vi "CNT State.vi"(7 "reset?":bool, 11 "Cross CSM Data":T1={"Name(\"\" to use uuid)"="CSM Tiny", "Current State"="UI: Refresh Buttons", "Arguments"="", "Source Message"={"‘State"="", "’Arguments"="", "’Error"={"status"=FALSE, "code"=0, "source"=""}}, "Source Module"="<end>", "Complete(T)/Start(F)"=TRUE, "LogType"=enum."State Change"}) -> (0 "Boolean":bool, 3 "Log String":string)   [LabVIEW 2017]
uses:
  _Support/Typedef/_CSM_GlobalLog_MSG.ctl
  _Support/Typedef/_CSM_Response Source Message.ctl
  _Support/Typedef/_CSM_GlobalLog_MSG_TYPE.ctl
  Communicable State Machine.lvlib
panel:
  in  "y":i64=2
  out "Map 3":variant=variant("CSM Tiny.DAQ: Break Continuous"=variant(i64 1), "CSM Tiny.DAQ: Close"=variant(i64 1), "CSM Tiny.DAQ: Configure"=variant(i64 1), "CSM Tiny.DAQ: Continuous Check"=variant(i64 188), "CSM Tiny.DAQ: Initialize"=variant(i64 1), "CSM Tiny.DAQ: Start"=variant(i64 1), "CSM Tiny.DAQ: Stop"=variant(i64 1), "CSM Tiny.Data"=variant(i64 95), "CSM Tiny.Data: Acquisite"=variant(i64 95), "CSM Tiny.UI: Refresh Buttons"=variant(i64 2))
  out "Map 2":variant=variant("CSM Tiny.DAQ: Break Continuous"=variant(u32 953145328), "CSM Tiny.DAQ: Close"=variant(u32 953145328), "CSM Tiny.DAQ: Configure"=variant(u32 953126122), "CSM Tiny.DAQ: Continuous Check"=variant(u32 953144928), "CSM Tiny.DAQ: Initialize"=variant(u32 953126122), "CSM Tiny.DAQ: Start"=variant(u32 953126122), "CSM Tiny.DAQ: Stop"=variant(u32 953145328), "CSM Tiny.Data"=variant(u32 953144928), "CSM Tiny.Data: Acquisite"=variant(u32 953144928), "CSM Tiny.UI: Refresh Buttons"=variant(u32 953145328))
  out "Map":variant=variant("CSM Tiny.DAQ: Break Continuous"=variant(i64 1), "CSM Tiny.DAQ: Close"=variant(i64 1), "CSM Tiny.DAQ: Configure"=variant(i64 1), "CSM Tiny.DAQ: Continuous Check"=variant(i64 192), "CSM Tiny.DAQ: Initialize"=variant(i64 1), "CSM Tiny.DAQ: Start"=variant(i64 1), "CSM Tiny.DAQ: Stop"=variant(i64 1), "CSM Tiny.Data"=variant(i64 97), "CSM Tiny.Data: Acquisite"=variant(i64 97), "CSM Tiny.UI: Refresh Buttons"=variant(i64 3))
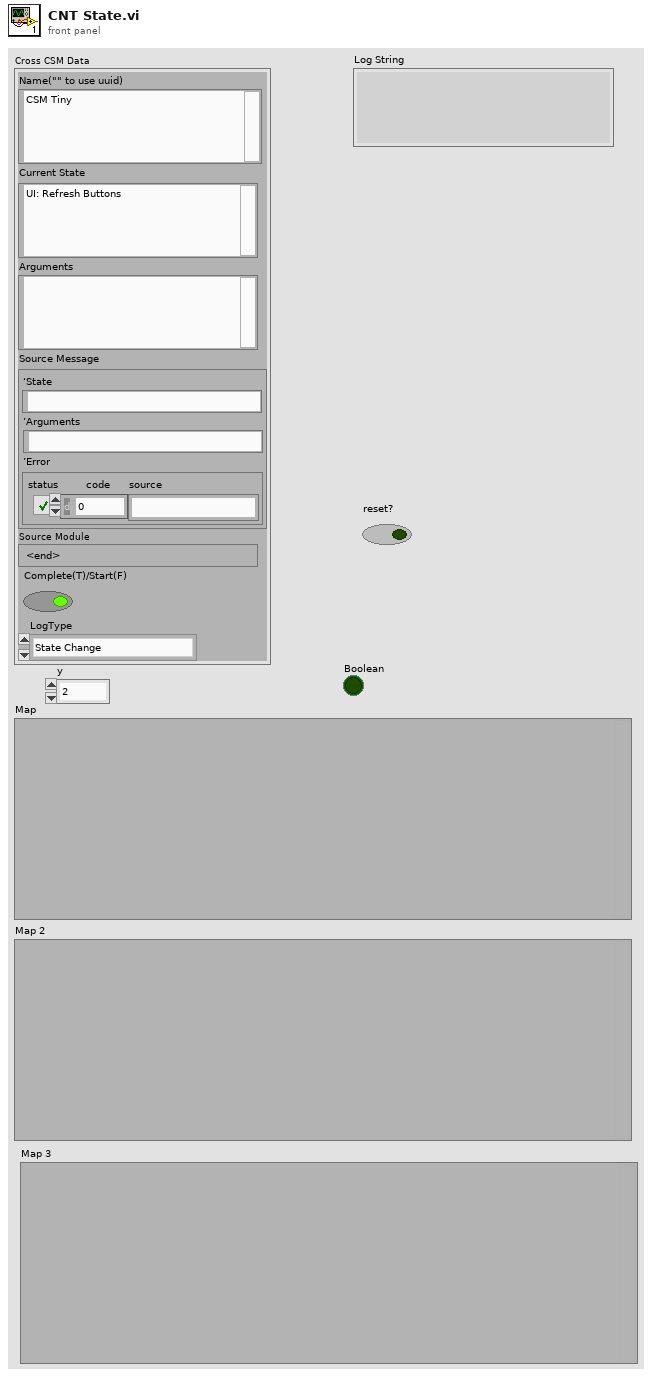
[diagram p1: front panel]
types:
  T1 = typedef "Communicable State Machine.lvlib/_CSM_GlobalLog_MSG.ctl" = cluster{"Name(\"\" to use uuid)":string, "Current State":string, "Arguments":string, "Source Message":T2, "Source Module":string, "Complete(T)/Start(F)":bool, "LogType":T3}
  T2 = typedef "Communicable State Machine.lvlib/_CSM_Response Source Message.ctl" = cluster{"‘State":string, "’Arguments":string, "’Error":errorcluster}
  T3 = typedef "Communicable State Machine.lvlib/_CSM_GlobalLog_MSG_TYPE.ctl" = enum16{"User Log", "State Change", "Status", "Interrupt", "Register", "Unregister", "Error Log", "Module Created", "Module Destroyed"}
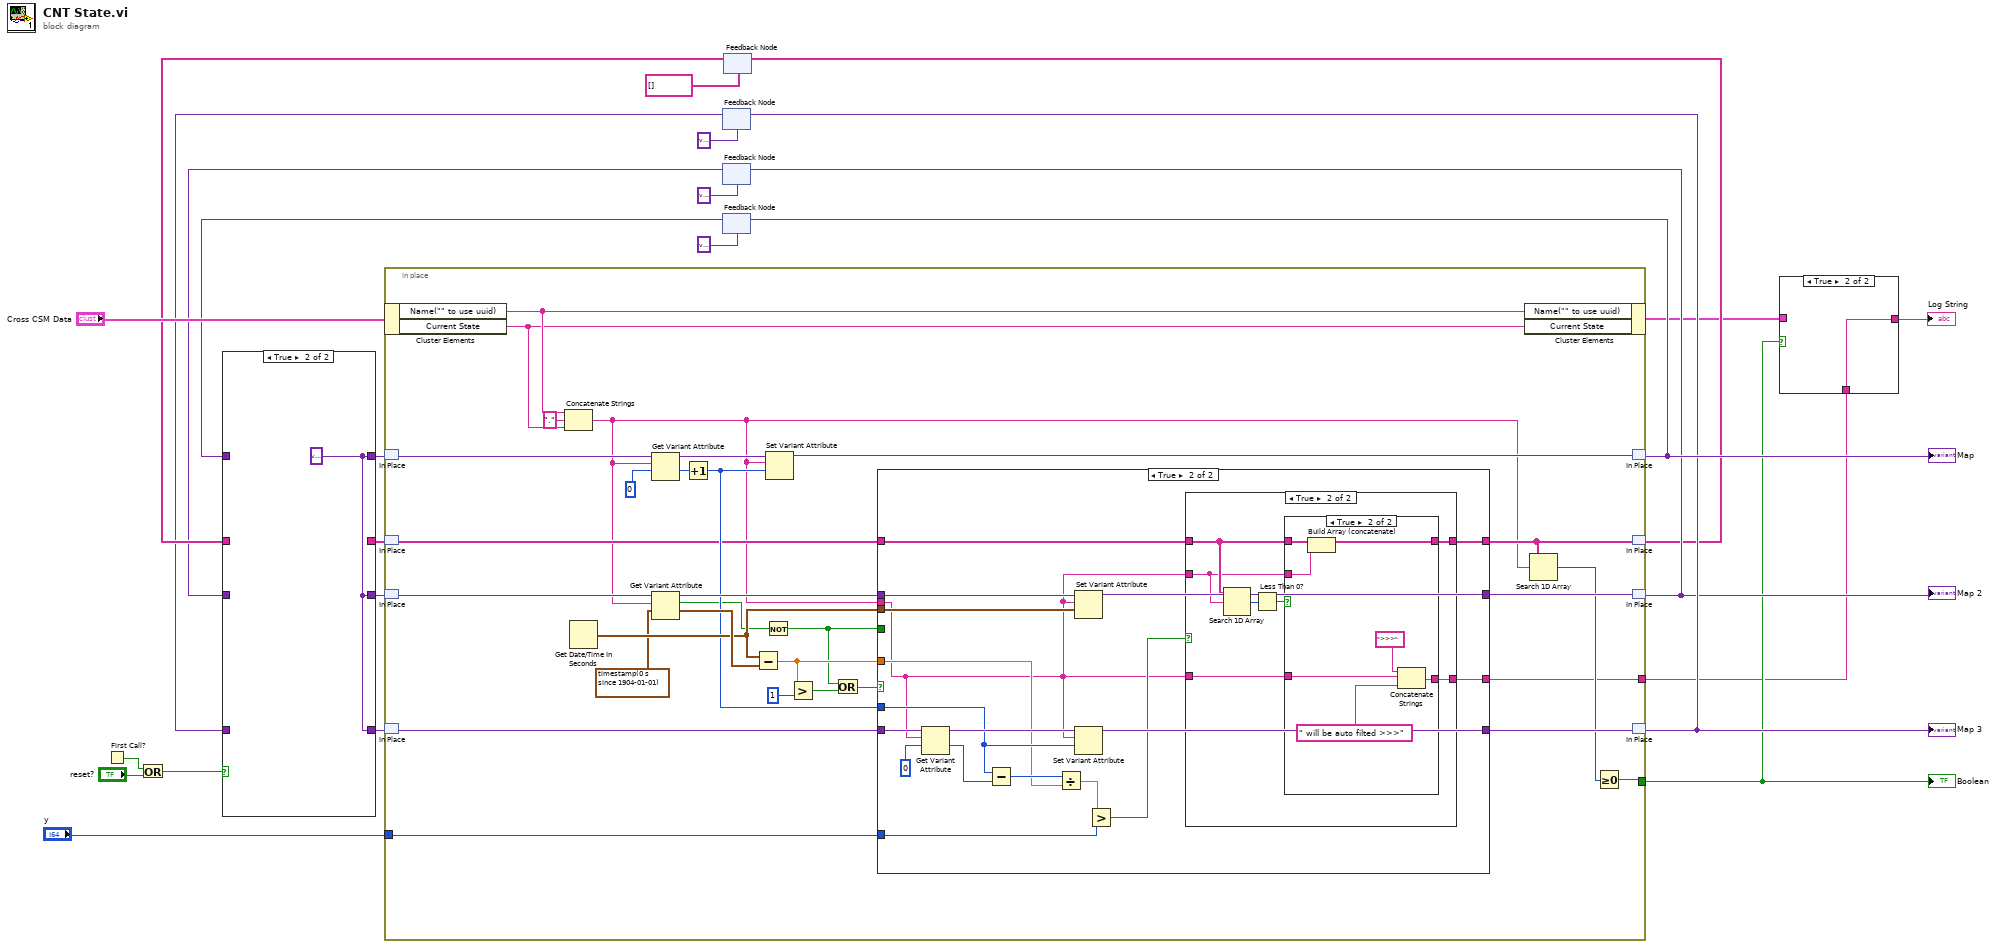
[diagram p0: block diagram]
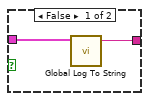
[diagram p3: hidden frame]
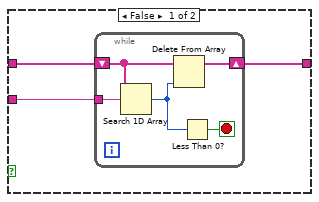
[diagram p5: hidden frame]
diagram:
  n1 = First Call?() -> (First Call?: T/F=w11:bool)
  n2 = Or(x=w11, y="reset?") -> (x .or. y?=w9:bool)
  n3 = feedback #1(variant) -> (w2:variant)
  n4 = feedback #2(variant) -> (w4:variant)
  n5 = feedback #3(variant) -> (w7:variant)
  n6 = feedback #4(string[] [] ("concatenated string")) -> (w5:string[])
  n7 = case shown="True" w9 {
    tunnel: [w29 w30] -> w8
    tunnel: w7 -> [w29 _]
    tunnel: [w28 _] -> w6
    tunnel: w5 -> [w28 _]
    tunnel: w4 -> [w27 _]
    tunnel: [w27 w30] -> w3
    tunnel: w2 -> [w26 _]
    tunnel: [w26 w30] -> w1
    frame False {
    }
    frame True {
      w30 = variant
    }
  }
  n8 = in-place {
    in-place-border: "y" -> [w40]
    in-place-border: [w35] -> w13
    in-place-border: [w33] -> w12
    n9 = in-place-cluster #5("Cross CSM Data") -> ("Name(\"\" to use uuid)"=w56:string, "Current State"=w55:string)
    n10 = in-place-match #6(w8) -> (w53:variant)
    n11 = in-place-match #7(w6) -> (w39:string[])
    n12 = in-place-match #8(w3) -> (w51:variant)
    n13 = in-place-match #9(w1) -> (w46:variant)
    n14 = Concatenate Strings(w56, "." ("string"), w55) -> (w36:string)
    n15 = Get Date/Time In Seconds() -> (seconds since 1Jan1904=w48:timestamp)
    n16 = Get Variant Attribute(Variant=w53, name=w36, default value (empty Variant)=i64 0 ("64bit integer")) -> (duplicate Variant=w58:variant, value=w59:i64)  [unwired: 1 in, 2 out]
    n17 = Get Variant Attribute(Variant=w51, name=w36, default value (empty Variant)=timestamp(0 s since 1904-01-01) ("current time")) -> (duplicate Variant=w52:variant, found=w42:bool, value=w49:timestamp)  [unwired: 1 in, 1 out]
    n18 = Increment(x=w59) -> (x+1=w44:i64)
    n19 = Subtract(x=w48, y=w49) -> (x-y=w38:dbl)
    n20 = Not(x=w42) -> (.not. x?=w32:bool)
    n21 = Set Variant Attribute(Variant=w58, name=w36, value=w44) -> (Variant out=w54:variant)  [unwired: 1 in, 2 out]
    n22 = Greater?(x=w38, y=u32 1) -> (0:w43:bool)
    n23 = Or(x=w32, y=w43) -> (x .or. y?=w41:bool)
    n24 = case shown="True" w41 {
      tunnel: w52 -> [w63 w81]
      tunnel: [w63 w80] -> w50
      tunnel: w48 -> [_ w79]
      tunnel: w46 -> [w62 w77]
      tunnel: [w62 w78] -> w45
      tunnel: w44 -> [_ w74]
      tunnel: w36 -> [_ w65]
      tunnel: w40 -> [_ w72]
      tunnel: w39 -> [w61 w71]
      tunnel: [w61 w70] -> w37
      tunnel: w38 -> [_ w66]
      tunnel: [_ w64] -> w33
      tunnel: w32 -> [_ _]
      frame False {
      }
      frame True {
        n25 = Get Variant Attribute(Variant=w77, name=w65, default value (empty Variant)=i64 0 ("64bit integer")) -> (duplicate Variant=w76:variant, value=w73:i64)  [unwired: 1 in, 2 out]
        n26 = Subtract(x=w74, y=w73) -> (x-y=w68:i64)
        n27 = Divide(x=w68, y=w66) -> (x/y=w67:dbl)
        n28 = Set Variant Attribute(Variant=w81, name=w65, value=w79) -> (Variant out=w80:variant)  [unwired: 1 in, 2 out]
        n29 = Set Variant Attribute(Variant=w76, name=w65, value=w74) -> (Variant out=w78:variant)  [unwired: 1 in, 2 out]
        n30 = Greater?(x=w67, y=w72) -> (0:w69:bool)
        n31 = case shown="True" w69 {
          tunnel: w71 -> [w83 w95]
          tunnel: [w82 w96] -> w70
          tunnel: w65 -> [w84 w94]
          tunnel: w65 -> [_ w91]
          tunnel: [_ w90] -> w64
          frame False {
            n32 = while {
              tunnel: w84 -> [w89]
              shift-right: [w87] -> w82
              shift-left: w83 -> [w88]
              stop <- w85 stop-if-true
              n33 = Search 1D Array(1D array=w88, element=w89) -> (index of element=w86:i32)  [unwired: 1 in]
              n34 = Delete From Array(array=w88, index=w86) -> (array with subset deleted=w87:string[])  [unwired: 1 in, 1 out]
              n35 = Less Than 0?(x=w86) -> (x < 0?=w85:bool)
            }
          }
          frame True {
            n36 = Search 1D Array(1D array=w95, element=w94) -> (index of element=w93:i32)  [unwired: 1 in]
            n37 = Less Than 0?(x=w93) -> (x < 0?=w92:bool)
            n38 = case shown="True" w92 {
              tunnel: [w97 w104] -> w96
              tunnel: w95 -> [w97 w103]
              tunnel: w94 -> [_ w102]
              tunnel: w91 -> [_ w101]
              tunnel: [_ w99] -> w90
              frame False {
              }
              frame True {
                n39 = Build Array (concatenate)(w103, w102) -> (w104:string[])
                n40 = Concatenate Strings(">>>" ("string"), w101, " will be auto filted >>>" ("string")) -> (w99:string)
              }
            }
          }
        }
      }
    }
    n41 = in-place-cluster #5("Name(\"\" to use uuid)"=w56, "Current State"=w55) -> (w15:T1)
    n42 = Search 1D Array(1D array=w37, element=w36) -> (index of element=w34:i32)  [unwired: 1 in]
    n43 = Greater Or Equal To 0?(x=w34) -> (x >= 0?=w35:bool)
    n44 = in-place-match #6(w54) -> (w23:variant)
    n45 = in-place-match #7(w37) -> (w16:string[])
    n46 = in-place-match #8(w50) -> (w19:variant)
    n47 = in-place-match #9(w45) -> (w20:variant)
  }
  "Map" <- w23
  "Map 2" <- w19
  "Map 3" <- w20
  "Boolean" <- w13
  n48 = feedback-in #1(w20) -> ()
  n49 = feedback-in #2(w19) -> ()
  n50 = feedback-in #3(w23) -> ()
  n51 = feedback-in #4(w16) -> ()
  n52 = case shown="True" w13 {
    tunnel: [w106 w107] -> w14
    tunnel: w15 -> [w105 _]
    tunnel: w12 -> [_ w107]
    frame False {
      n53 = call "Global Log To String.vi"("Log"=w105) -> ("Log String"=w106:string)  [unwired: 9 in]
    }
    frame True {
    }
  }
  "Log String" <- w14
